vi "AVI-Validate playback parameters.vi"() -> (1 "Zero value detected":bool, 3 "index of element":i32)   [LabVIEW 2020]
uses:
  Functional Imaging Viewer/SubVIs/Experiment header interface/Typedefs/Header file interface module functions enum.ctl
  Functional Imaging Viewer/SubVIs/Experiment header interface/Typedefs/Header file sections.ctl
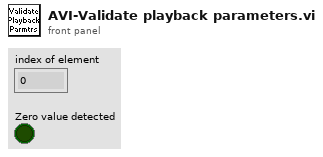
[diagram p1: front panel]
types:
  T1 = typedef "Header file sections.ctl" = enum16{"ALL SECTIONS", "LOGIN", "GLOBAL PARAMETERS", "CALIBRATION DATA", "IMAGING MODES", "TIME SERIES", "MOTOR Z-STACK", "AOL Z-STACK", "FUNCTIONAL IMAGING", "VOLUME IMAGING", "MOVEMENT CORRECTION", "CALIBRATION", "STATISTICS", "BIOLOGY INFORMATION"}
  T2 = typedef "Header file interface module functions enum.ctl" = enum16{"Load experiment header file", "Save experiment header file", "Clear stored values", "Read stored values", "Update specific value in memory", "Update values in memory"}
  T3 = typedef "Header parameters cluster-ALL.ctl" = cluster{"LOGIN":T4, "GLOBAL PARAMETERS":T5, "IMAGING MODES":T7, "TIME SERIES":T8, "MOTOR Z-STACK ":T11, "AOL Z-STACK":T12, "FUNCTIONAL IMAGING":T13, "VOLUME IMAGING":T13, "MOVEMENT CORRECTION":T17, "CALIBRATION":T19, "STATISTICS":T20, "BIOLOGY INFORMATION":T21, "Calibration Data":T22}
  T4 = typedef "Header params -Login.ctl" = cluster{"User":string, "Profile":string, "Software Version":string, "Experiment Date Time":timestamp}
  T5 = typedef "Header params-Global Parameters.ctl" = cluster{"MicroscopeID":string, "Microscope Type":string, "Objective":string, "Field of View (um)":dbl, "Fill time (us)":dbl, "Experiment Type":T6, "Stimuli Trigger":bool, "Speed Logging":bool}
  T6 = typedef "Experiment Type.ctl" = enum16{"In vivo", "In vitro", "Testing", "Calibration", "Other"}
  T7 = typedef "Header params-Imaging Modes.ctl" = cluster{"Time Series":bool, "Motor Zstack":bool, "AOL Zstack":bool, "Functional Imaging":bool, "Volume Imaging":bool}
  T8 = typedef "Header params-Time Series.ctl" = cluster{"Basic Image meta data":T9, "AOL z":dbl}
  T9 = typedef "Header params-Basic image meta data.ctl" = cluster{"Wavelength (nm)":dbl, "# averaged frames":dbl, "laser power (%)":dbl, "Pockels":dbl, "pixel dwell time (us)":dbl, "pmt 1":dbl, "pmt 2":dbl, "back apperture":dbl, "zoom":dbl, "field of view":dbl, "Frame Size":T10, "AOL x centre":dbl, "AOL y centre":dbl, "Stage x position":dbl, "Stage y position":dbl, "Stage z position":dbl}
  T10 = typedef "Frame Size.ctl" = u16
  T11 = typedef "Header params-Motor Z-stack.ctl" = cluster{"Hdr Basic Image meta data":T9, "Z Start":dbl, "Z Stop":dbl, "No of Planes":i32, "Laser Power (%) at Z Start":dbl, "Laser Power (%) at Z Stop":dbl}
  T12 = typedef "Header params-AOL Z-stack.ctl" = cluster{"Hdr Basic Image meta data":T9, "Z Start":dbl, "Z Stop":dbl, "No of Planes":i32, "Laser Power (%) at Z Start":dbl, "Laser Power (%) at Z Stop":dbl}
  T13 = typedef "Header params-Functional Imaging.ctl" = cluster{"Functional Mode":T14, "Variable Length":bool, "Variable Resolution":bool, "Pockels Modulation":bool, "Stimuli Trigger":bool, "Cool down enabled":bool, "AOL Mode":T15, "Plane Mode":T16, "Miniscan Dwell time per pixel (us)":dbl, "poi dwell time":dbl, "Number of trials":dbl, "Number of cycles":dbl, "Number of pois":dbl, "Number of miniscans":dbl, "Number of pixels in miniscan":dbl, "Rectangle ROI length":dbl, "Rectangle ROI height":dbl, "Frame rate (fps)":dbl, "Acquisition Length":dbl, "video length (sec)":dbl, "Stimuli delay (sec)":dbl, "Cool down time (sec)":dbl, "Basic Image meta data":T9, "Z Start (um)":dbl, "Z Stop (um)":dbl}
  T14 = typedef "Functional Mode.ctl" = enum16{"Point", "Line", "Patch", "Plane", "Volume"}
  T15 = typedef "AOL modes.ctl" = enum16{"Raster", "Structural", "Pointing", "Mini Scan", "Alignment"}
  T16 = typedef "Plane Mode.ctl" = u16
  T17 = typedef "Header params-Movement correction.ctl" = cluster{"Movement Correction":bool, "Axial Reference":bool, "Reference Source":T18, "Full Frame Size":dbl, "Reference Field of View":dbl, "Reference Zoom":dbl, "Reference dwell time (us)":dbl, "Reference X Pixels":dbl, "Reference Y Pixels":dbl, "Number of Z lines":dbl, "Size of Z pixels":dbl, "Axial Pixels":dbl, "Ignore Z lines":dbl, "Reference Scan Cycles":dbl, "Reference Threshold XY":dbl, "Reference Threshold Z":dbl, "Reference Average XY":dbl, "Reference Average Z":dbl, "Proportional Scale":dbl, "Integral Scale":dbl, "Proportional Scale Z":dbl, "Integral Scale Z":dbl, "Diff Threshold":dbl, "Diff Threshold Z":dbl, "Sliding Average":bool, "Reference count reset enabled":bool, "Scan Interval (ms)":dbl, "Ref Plot Refresh Rate (ms)":dbl}
  T18 = typedef "Reference source.ctl" = enum16{"Green channel", "Red channel"}
  T19 = typedef "Header params-Calibration Setup.ctl" = cluster{"Pockels Calibration File":path, "Calibration_ini file":path, "Setup_ini file":path}
  T20 = typedef "Header params-statistics.ctl" = cluster{"Z-stack duration (sec)":dbl, "Number of acquired data-points":dbl, "Acquisition time (ms)":dbl, "Number of acquired frames":dbl, "Intertrial times":dbl[]}
  T21 = typedef "Biology Information.ctl" = cluster{"Animal Code or Name":string, "Animal DoB":string, "Animal Age":string, "Animal Sex":string, "Animal Weight":string, "Date of Injection":string, "Date of Implant":string, "Site of Injection":string, "Animal Ear Notch":string, "AAV constructs":string, "Genetic background":string, "Optical reporter":string, "Region of brain imaged":string, "Other \ncomments":string}
  T22 = typedef "Header params-calibration data.ctl" = cluster{"Objective Name":string, "Calibration Wavelength":dbl, "Sum X":dbl, "Sum Y":dbl, "Diff X":dbl, "Diff Y":dbl, "Distortion Correction":dbl, " Z norm to um Scaling":dbl, " X norm to um Scaling":dbl}
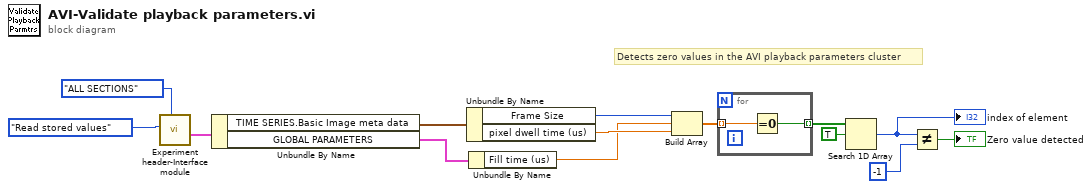
[diagram p0: block diagram]
diagram:
  # "Detects zero values in the AVI playback parameters cluster"
  n1 = call "Experiment header-Interface module.vi"("Header file sections"=Header_file_sections."ALL SECTIONS", "Function"=Header_file_interface_module_functions_enum."Read stored values") -> ("All header parameters out"=w4:T3)  [unwired: 8 in, 1 out]
  n2 = Unbundle By Name(w4) -> ("TIME SERIES.Basic Image meta data"=w2:T9, "GLOBAL PARAMETERS"=w1:T5)
  n3 = Unbundle By Name(w2) -> ("Frame Size"=w7:T10, "pixel dwell time (us)"=w8:dbl)
  n4 = Unbundle By Name(w1) -> ("Fill time (us)"=w3:dbl)
  n5 = Build Array(w7, w3, w8) -> (w9:dbl[])
  n6 = for {
    tunnel: w9 -> [w16] mode=indexing
    tunnel: [w15] -> w10 mode=indexing
    n7 = Equal To 0?(x=w16) -> (x = 0?=w15:bool)
  }
  n8 = Search 1D Array(1D array=w10, element=TRUE) -> (index of element=w14:i32)  [unwired: 1 in]
  "index of element" <- w14
  n9 = Not Equal?(x=w14, y=-1) -> (x != y?=→"Zero value detected":bool)
